vi "Get Resource ID.vi"(4 "SPI in":refnum<class "SPI.lvclass">) -> (7 "Resource ID":string)   [LabVIEW 2024, in "CTI.lvlib" / "SPI.lvclass"]
uses:
  SPI.lvclass
  SPI.lvclass/SPI.ctl
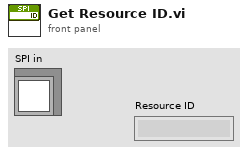
[diagram p1: front panel]
types:
  T1 = typedef "CTI.lvlib/SPI Number.ctl" = i8
  T2 = typedef "CTI.lvlib/GPIO Number.ctl" = i8
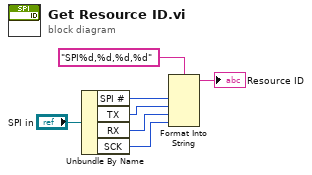
[diagram p0: block diagram]
diagram:
  n1 = Unbundle By Name("SPI in") -> ("SPI #"=w5:T1, "TX"=w3:T2, "RX"=w1:T2, "SCK"=w2:T2)
  n2 = Format Into String(format string="SPI%d,%d,%d,%d", w5, w3, w1, w2) -> (resulting string=→"Resource ID":string)  [unwired: 2 in, 1 out]
